vi "Zero IMU.vi"   [LabVIEW 2017]
uses:
  Robot Global Data.vi
  navX.Library.v2/navX Library v2/navX Library v2.lvlib
types:
  T1 = typedef "navX Library v2.lvlib/Z900_navX_DeviceTypeDef.ctl" = cluster{"Interface":cluster{"Protocol":T2, "Update Rate (4Hz-60Hz)":u8, "navX Open TypeDef":variant}, "Notify Packet":refnum<notifier>, "Loop VI Refnum":refnum<vi>, "Ready to Close Occurrence Refnum":refnum<k4>}
  T2 = typedef "navX Library v2.lvlib/Z900_navX_ProtocolTypeDef.ctl" = enum16{"SERIAL", "I2C", "SPI"}
  T3 = cluster{"Yaw":dbl, "Roll":dbl, "Pitch":dbl, "Heading":dbl, "Fused Heading":dbl}
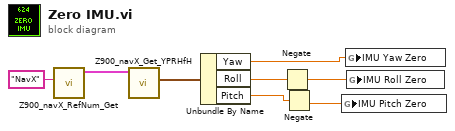
[diagram p0: block diagram]
diagram:
  n1 = call "Z900_navX_RefNum_Get.vi"("refnum name"="NavX") -> ("navX Device"=w8:T1)  [unwired: 9 in, 1 out]
  n2 = call "Z900_navX_Get_YPRHfH.vi"("navX Device"=w8) -> ("YRPHfH"=w6:T3)  [unwired: 7 in, 3 out]
  n3 = Unbundle By Name(w6) -> ("Yaw"=w3:dbl, "Roll"=w5:dbl, "Pitch"=w4:dbl)
  n4 = Negate(x=w5) -> (-x=w2:dbl)
  n5 = Negate(x=w4) -> (-x=w1:dbl)
  n6 = global write "Robot Global Data.vi" "IMU Pitch Zero"(w1) -> ()
  n7 = global write "Robot Global Data.vi" "IMU Yaw Zero"(w3) -> ()
  n8 = global write "Robot Global Data.vi" "IMU Roll Zero"(w2) -> ()
